vi "Cluster8ToCluster67.vi"(0 "簇":T2, 1 "NAM":string, 2 "TDN":string, 3 "PROD":string, 4 "CALD":string, 5 "REV":string) -> (17 "输出簇":T1)   [LabVIEW 2019]
uses:
  Test_data.ctl
  Test_load.ctl
  Hardness_test.ctl
  Cluster67.ctl
  TEST.lvclass
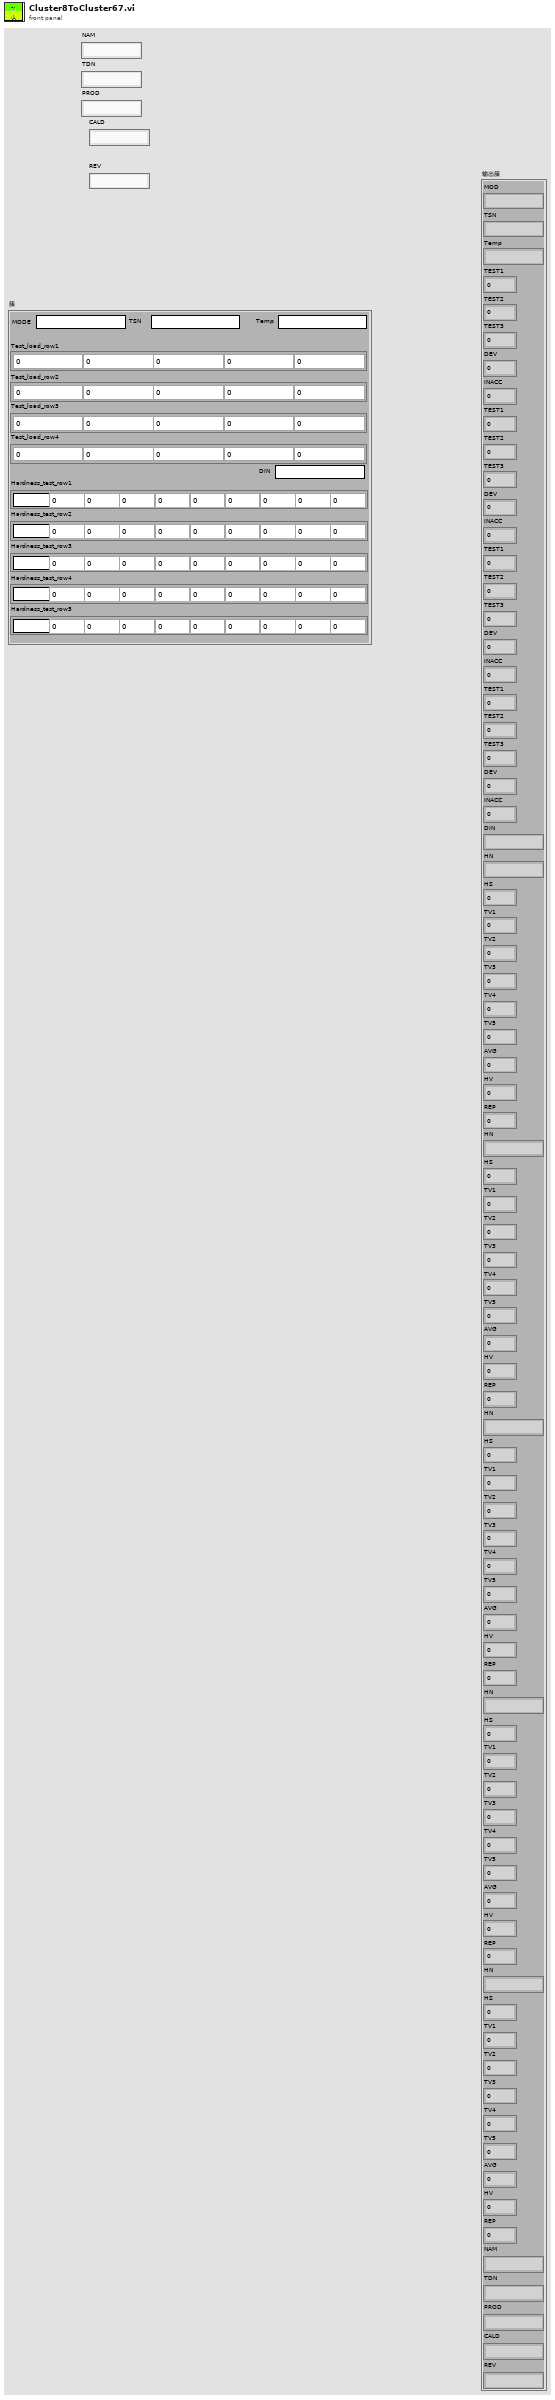
[diagram p1: front panel]
types:
  T1 = typedef "TEST.lvclass/Cluster67.ctl" = cluster{"MOD":string, "TSN":string, "Temp":string, "TEST1":sgl, "TEST2":sgl, "TEST3":sgl, "DEV":sgl, "INACC":sgl, "TEST1":sgl, "TEST2":sgl, "TEST3":sgl, "DEV":sgl, "INACC":sgl, "TEST1":sgl, "TEST2":sgl, "TEST3":sgl, "DEV":sgl, "INACC":sgl, "TEST1":sgl, "TEST2":sgl, "TEST3":sgl, "DEV":sgl, "INACC":sgl, "DIN":string, "HN":string, "HS":sgl, "TV1":sgl, "TV2":sgl, "TV3":sgl, "TV4":sgl, "TV5":sgl, "AVG":sgl, "HV":sgl, "REP":sgl, "HN":string, "HS":sgl, "TV1":sgl, "TV2":sgl, "TV3":sgl, "TV4":sgl, "TV5":sgl, "AVG":sgl, "HV":sgl, "REP":sgl, "HN":string, "HS":sgl, "TV1":sgl, "TV2":sgl, "TV3":sgl, "TV4":sgl, "TV5":sgl, "AVG":sgl, "HV":sgl, "REP":sgl, "HN":string, "HS":sgl, "TV1":sgl, "TV2":sgl, "TV3":sgl, "TV4":sgl, "TV5":sgl, "AVG":sgl, "HV":sgl, "REP":sgl, "HN":string, "HS":sgl, "TV1":sgl, "TV2":sgl, "TV3":sgl, "TV4":sgl, "TV5":sgl, "AVG":sgl, "HV":sgl, "REP":sgl, "NAM":string, "TDN":string, "PROD":string, "CALD":string, "REV":string}
  T2 = typedef "TEST.lvclass/Test_data.ctl" = cluster{"MODE":string, "TSN":string, "Temp":string, "Test_load_row1":T3, "Test_load_row2":T3, "Test_load_row3":T3, "Test_load_row4":T3, "DIN":string, "Hardness_test_row1":T4, "Hardness_test_row2":T4, "Hardness_test_row3":T4, "Hardness_test_row4":T4, "Hardness_test_row5":T4}
  T3 = typedef "TEST.lvclass/Test_load.ctl" = cluster{"TEST1":sgl, "TEST2":sgl, "TEST3":sgl, "DEV":sgl, "INACC":sgl}
  T4 = typedef "TEST.lvclass/Hardness_test.ctl" = cluster{"HN":string, "HS":sgl, "TV1":sgl, "TV2":sgl, "TV3":sgl, "TV4":sgl, "TV5":sgl, "AVG":sgl, "HV":sgl, "REP":sgl}
  T5 = cluster{"MODE":string, "TSN":string, "Temp":string, "TEST1":sgl, "TEST2":sgl, "TEST3":sgl, "DEV":sgl, "INACC":sgl, "TEST1":sgl, "TEST2":sgl, "TEST3":sgl, "DEV":sgl, "INACC":sgl, "TEST1":sgl, "TEST2":sgl, "TEST3":sgl, "DEV":sgl, "INACC":sgl, "TEST1":sgl, "TEST2":sgl, "TEST3":sgl, "DEV":sgl, "INACC":sgl, "DIN":string, "HN":string, "HS":sgl, "TV1":sgl, "TV2":sgl, "TV3":sgl, "TV4":sgl, "TV5":sgl, "AVG":sgl, "HV":sgl, "REP":sgl, "HN":string, "HS":sgl, "TV1":sgl, "TV2":sgl, "TV3":sgl, "TV4":sgl, "TV5":sgl, "AVG":sgl, "HV":sgl, "REP":sgl, "HN":string, "HS":sgl, "TV1":sgl, "TV2":sgl, "TV3":sgl, "TV4":sgl, "TV5":sgl, "AVG":sgl, "HV":sgl, "REP":sgl, "HN":string, "HS":sgl, "TV1":sgl, "TV2":sgl, "TV3":sgl, "TV4":sgl, "TV5":sgl, "AVG":sgl, "HV":sgl, "REP":sgl, "HN":string, "HS":sgl, "TV1":sgl, "TV2":sgl, "TV3":sgl, "TV4":sgl, "TV5":sgl, "AVG":sgl, "HV":sgl, "REP":sgl, "NAM":string, "TDN":string, "PROD":string, "CALD":string, "REV":string}
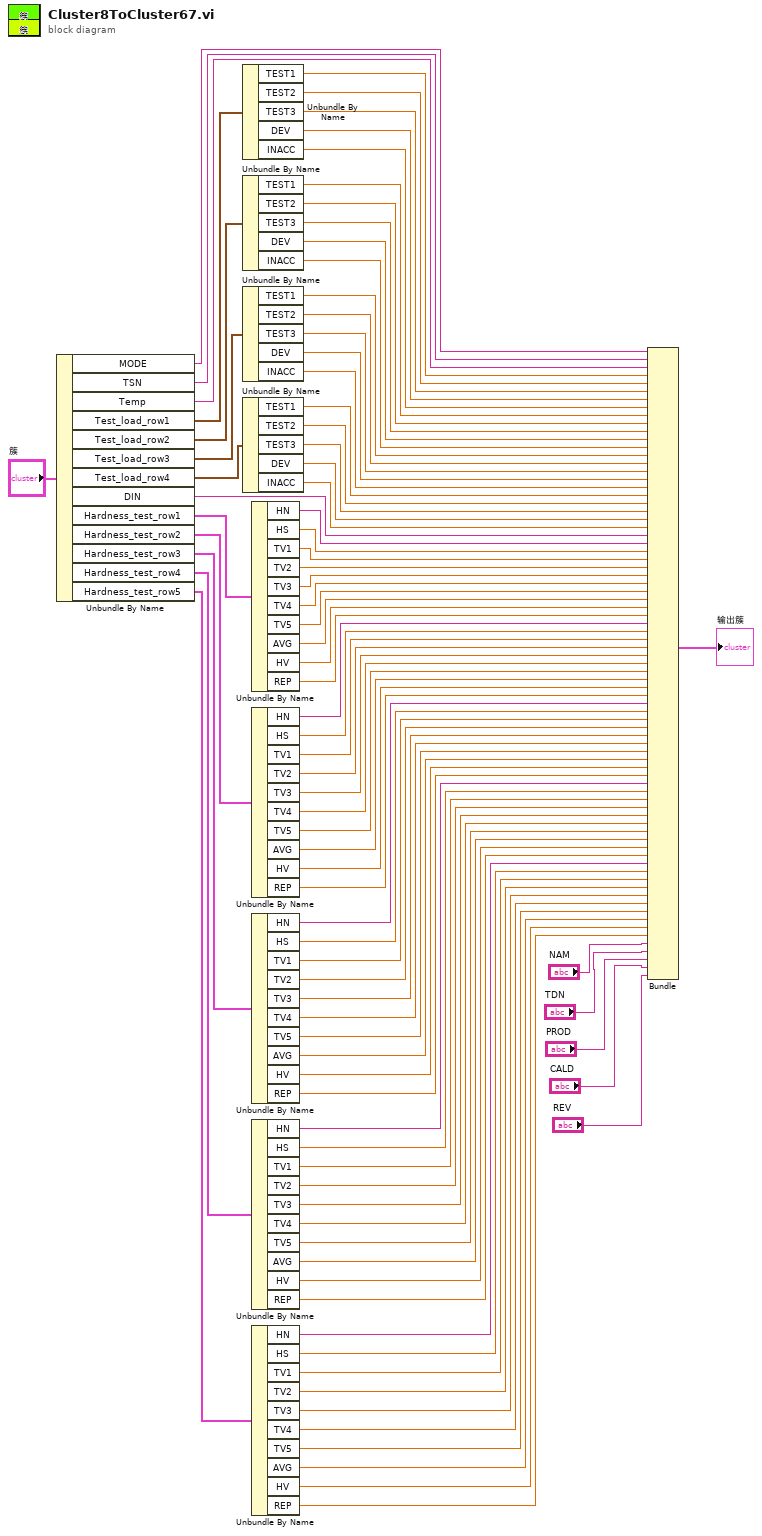
[diagram p0: block diagram]
diagram:
  n1 = Unbundle By Name("簇") -> ("MODE"=w9:string, "TSN"=w31:string, "Temp"=w30:string, "Test_load_row1"=w89:T3, "Test_load_row2"=w88:T3, "Test_load_row3"=w87:T3, "Test_load_row4"=w32:T3, "DIN"=w7:string, "Hardness_test_row1"=w37:T4, "Hardness_test_row2"=w36:T4, "Hardness_test_row3"=w35:T4, "Hardness_test_row4"=w34:T4, "Hardness_test_row5"=w33:T4)
  n2 = Unbundle By Name(w89) -> ("TEST1"=w29:sgl, "TEST2"=w28:sgl, "TEST3"=w27:sgl, "DEV"=w26:sgl, "INACC"=w25:sgl)
  n3 = Unbundle By Name(w88) -> ("TEST1"=w24:sgl, "TEST2"=w23:sgl, "TEST3"=w22:sgl, "DEV"=w21:sgl, "INACC"=w20:sgl)
  n4 = Unbundle By Name(w87) -> ("TEST1"=w19:sgl, "TEST2"=w18:sgl, "TEST3"=w17:sgl, "DEV"=w16:sgl, "INACC"=w15:sgl)
  n5 = Unbundle By Name(w32) -> ("TEST1"=w14:sgl, "TEST2"=w13:sgl, "TEST3"=w12:sgl, "DEV"=w11:sgl, "INACC"=w10:sgl)
  n6 = Unbundle By Name(w37) -> ("HN"=w8:string, "HS"=w86:sgl, "TV1"=w85:sgl, "TV2"=w84:sgl, "TV3"=w83:sgl, "TV4"=w82:sgl, "TV5"=w81:sgl, "AVG"=w80:sgl, "HV"=w79:sgl, "REP"=w78:sgl)
  n7 = Unbundle By Name(w36) -> ("HN"=w77:string, "HS"=w76:sgl, "TV1"=w75:sgl, "TV2"=w74:sgl, "TV3"=w73:sgl, "TV4"=w72:sgl, "TV5"=w71:sgl, "AVG"=w70:sgl, "HV"=w69:sgl, "REP"=w68:sgl)
  n8 = Unbundle By Name(w35) -> ("HN"=w67:string, "HS"=w66:sgl, "TV1"=w65:sgl, "TV2"=w64:sgl, "TV3"=w63:sgl, "TV4"=w62:sgl, "TV5"=w61:sgl, "AVG"=w60:sgl, "HV"=w59:sgl, "REP"=w58:sgl)
  n9 = Unbundle By Name(w34) -> ("HN"=w57:string, "HS"=w56:sgl, "TV1"=w55:sgl, "TV2"=w54:sgl, "TV3"=w53:sgl, "TV4"=w52:sgl, "TV5"=w51:sgl, "AVG"=w50:sgl, "HV"=w49:sgl, "REP"=w48:sgl)
  n10 = Unbundle By Name(w33) -> ("HN"=w47:string, "HS"=w46:sgl, "TV1"=w45:sgl, "TV2"=w44:sgl, "TV3"=w43:sgl, "TV4"=w42:sgl, "TV5"=w41:sgl, "AVG"=w40:sgl, "HV"=w39:sgl, "REP"=w38:sgl)
  n11 = Bundle("MODE"=w9, "TSN"=w31, "Temp"=w30, "TEST1"=w29, "TEST2"=w28, "TEST3"=w27, "DEV"=w26, "INACC"=w25, "TEST1"=w24, "TEST2"=w23, "TEST3"=w22, "DEV"=w21, "INACC"=w20, "TEST1"=w19, "TEST2"=w18, "TEST3"=w17, "DEV"=w16, "INACC"=w15, "TEST1"=w14, "TEST2"=w13, "TEST3"=w12, "DEV"=w11, "INACC"=w10, "DIN"=w7, "HN"=w8, "HS"=w86, "TV1"=w85, "TV2"=w84, "TV3"=w83, "TV4"=w82, "TV5"=w81, "AVG"=w80, "HV"=w79, "REP"=w78, "HN"=w77, "HS"=w76, "TV1"=w75, "TV2"=w74, "TV3"=w73, "TV4"=w72, "TV5"=w71, "AVG"=w70, "HV"=w69, "REP"=w68, "HN"=w67, "HS"=w66, "TV1"=w65, "TV2"=w64, "TV3"=w63, "TV4"=w62, "TV5"=w61, "AVG"=w60, "HV"=w59, "REP"=w58, "HN"=w57, "HS"=w56, "TV1"=w55, "TV2"=w54, "TV3"=w53, "TV4"=w52, "TV5"=w51, "AVG"=w50, "HV"=w49, "REP"=w48, "HN"=w47, "HS"=w46, "TV1"=w45, "TV2"=w44, "TV3"=w43, "TV4"=w42, "TV5"=w41, "AVG"=w40, "HV"=w39, "REP"=w38, "NAM"="NAM", "TDN"="TDN", "PROD"="PROD", "CALD"="CALD", "REV"="REV") -> (→"输出簇":T5)  [unwired: 1 in]
